vi "Plugin.Set Debug Flags.vi"(10 "Debug Flags":refnum<class "Debug Flags.lvclass">, 11 "Plugin in":refnum<class "Plugin.lvclass">) -> (3 "Plugin out":refnum<class "Plugin.lvclass">)   [LabVIEW 2017, in "DSF.Engine.lvlib" / "Plugin.lvclass"]
uses:
  Plugin.lvclass
  Debug/Debug Flags.lvclass
  Plugin.lvclass/Plugin.ctl
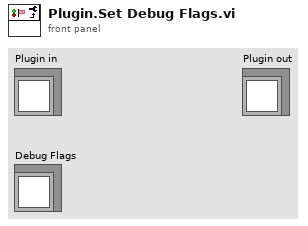
[diagram p1: front panel]
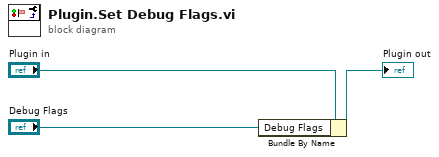
[diagram p0: block diagram]
diagram:
  n1 = Bundle By Name(cluster="Plugin in", "Debug Flags"="Debug Flags") -> (→"Plugin out":refnum<class "Plugin.lvclass">)
